vi "运维调试.vi"() -> ()   [LabVIEW 2016]
uses:
  <vilib>/Utility/miscctls.llb/LVPointTypeDef.ctl
  PLC/PLC.lvlib
  API/CodCr/CodCr.lvlib
panel:
  in  "运维调试单选按钮":T1(xcontrol)
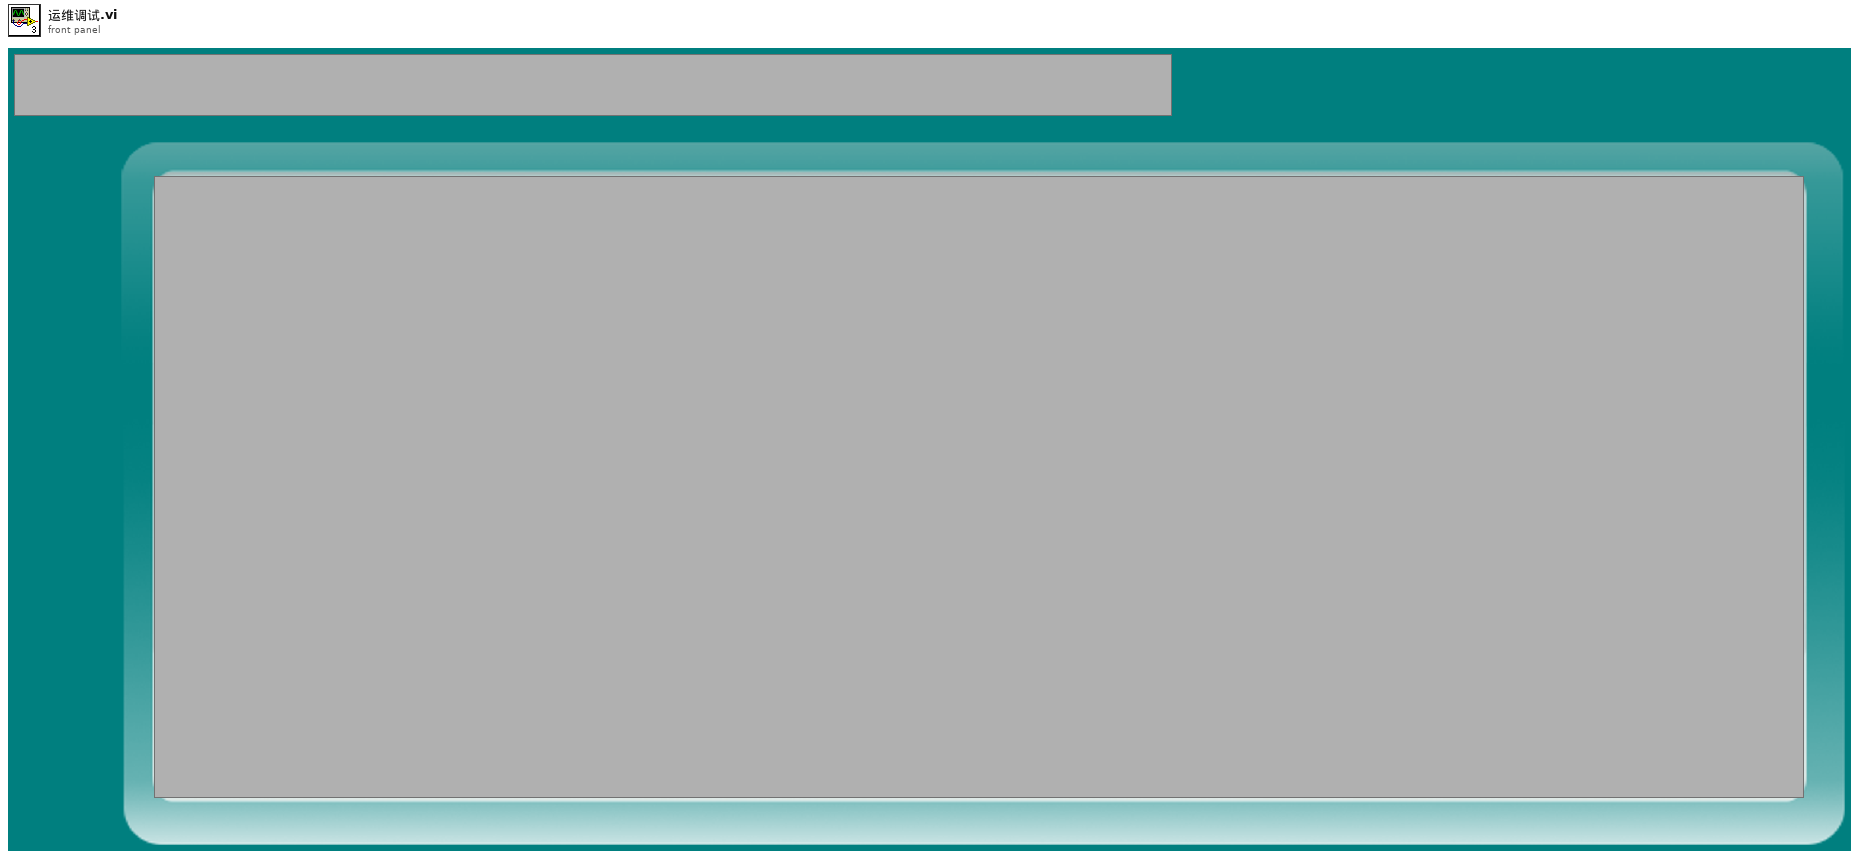
[diagram p1: front panel]
types:
  T1 = enum16{"采配水", "CODmn", "CODCr", "氨氮", "总磷总氮", "多参数", "质控单元", "其他"}
  T2 = typedef "LVPointTypeDef.ctl" = cluster{"Horizontal":i16, "Vertical":i16}
  T3 = enum32{"Bad", "Idle", "Run top level", "Running"}
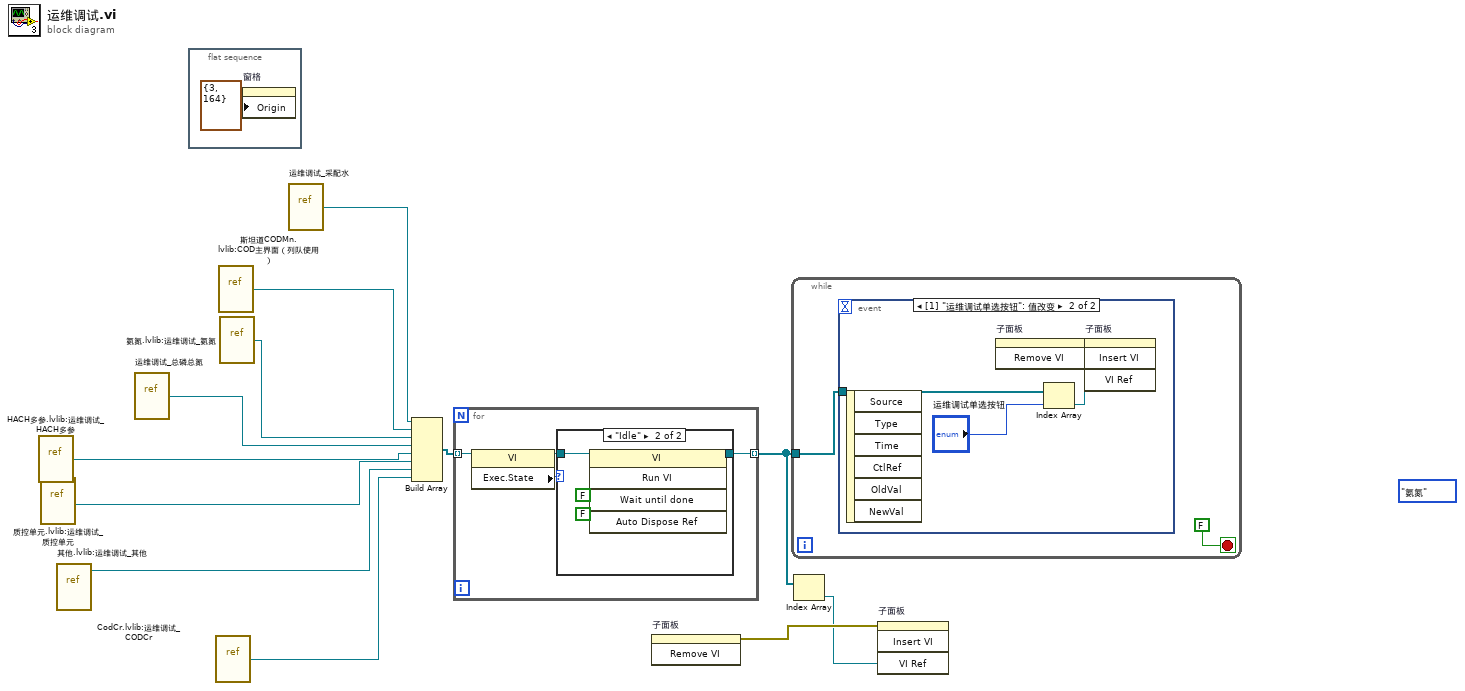
[diagram p0: block diagram]
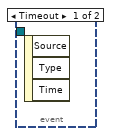
[diagram p3: hidden frame]
diagram:
  (unwired) T1."氨氮" ("运维调试单选按钮")
  n1 = vi-ref "HACH多参.lvlib:运维调试_HACH多参.vi"() -> (w5:refnum<vi>)
  n2 = vi-ref "质控单元.lvlib:运维调试_质控单元.vi"() -> (w4:refnum<vi>)
  n3 = vi-ref "其他.lvlib:运维调试_其他.vi"() -> (w3:refnum<vi>)
  n4 = vi-ref "运维调试_总磷总氮.vi"() -> (w1:refnum<vi>)
  n5 = flat-sequence {
    frame #0 {
      n6 = property on="窗格" class="Pane"("Origin"=T2 {"Horizontal"=3, "Vertical"=164} ("原点")) -> ()  [unwired: 2 in, 2 out]
    }
  }
  n7 = vi-ref "CodCr.lvlib:运维调试_CODCr.vi"() -> (w6:refnum<vi>)
  n8 = vi-ref "斯坦道CODMn.lvlib:COD主界面（列队使用）.vi"() -> (w7:refnum<vi>)
  n9 = vi-ref "氨氮.lvlib:运维调试_氨氮.vi"() -> (w2:refnum<vi>)
  n10 = vi-ref "运维调试_采配水.vi"() -> (w8:refnum<vi>)
  n11 = Build Array(w8, w7, w2, w1, w5, w4, w3, w6) -> (w9:refnum<vi>[])
  n12 = for {
    tunnel: w9 -> [w17] mode=indexing
    tunnel: [w14] -> w11 mode=indexing
    n13 = property class="VI"(reference=w17) -> (reference out=w15:refnum<vi>, "Exec.State"=w16:T3)  [unwired: 1 in, 1 out]
    n14 = case shown="\"Idle\"" w16 {
      tunnel: w15 -> [w18 w20]
      tunnel: [w18 w19] -> w14
      frame "Bad", Default {
      }
      frame "Idle" {
        n15 = invoke class="VI" method="Run VI"(reference=w20, "Wait until done"=FALSE ("结束前等待"), "Auto Dispose Ref"=FALSE ("自动销毁引用")) -> (reference out=w19:refnum<vi>)  [unwired: 2 in, 4 out]
      }
    }
  }
  n16 = invoke on="子面板" class="SubPnl" method="Remove VI"() -> (error out=w12:errorcluster)  [unwired: 3 in, 2 out]
  n17 = while {
    tunnel: w11 -> [w23]
    stop <- FALSE stop-if-true
    n18 = event shown="[1] \"运维调试单选按钮\": 值改变" {
      selector: _ -> [_ _]
      dyn-events: _ -> [_ _]
      timeout: _ -> [_ _]
      tunnel: w23 -> [_ w26]
      event Timeout {
        n19 = event-data() -> ()  [unwired: 1 in, 3 out]
      }
      event "运维调试单选按钮": Value Change {
        n20 = event-data() -> ()  [unwired: 1 in, 6 out]
        n21 = invoke on="子面板" class="SubPnl" method="Remove VI"() -> (error out=w28:errorcluster)  [unwired: 3 in, 2 out]
        n22 = Index Array(array=w26, index="运维调试单选按钮") -> (element=w25:refnum<vi>)
        n23 = invoke on="子面板" class="SubPnl" method="Insert VI"(error in=w28, "VI Ref"=w25) -> ()  [unwired: 2 in, 4 out]
      }
    }
  }
  n24 = Index Array(array=w11) -> (element=w10:refnum<vi>)  [unwired: 1 in]
  n25 = invoke on="子面板" class="SubPnl" method="Insert VI"(error in=w12, "VI Ref"=w10) -> ()  [unwired: 2 in, 4 out]
